vi "Default Instrument Setup.vi"(8 "error in (no error)":errorcluster, 11 "VISA resource name":refnum<visa-resource-name>) -> (0 "error out":errorcluster, 3 "VISA resource name out":refnum<visa-resource-name>)   [LabVIEW 2016, in "Andeen-Hagerling 2700.lvlib"]
doc: "This Utility VI sends a default command string to the instrument whenever a new VISA session is opened, or the instrument is reset. Use this VI as a subVI for the Initialize and Reset VIs. Altering this VI could cause these two VIs to operate incorrectly.\n\nThis VI configures the bridge for performing programmatic control. This includes turning off serial echo, labels, and setting error messages to numeric code, and turning on the Sample Swtich field."
uses:
  Andeen-Hagerling 2700.lvlib
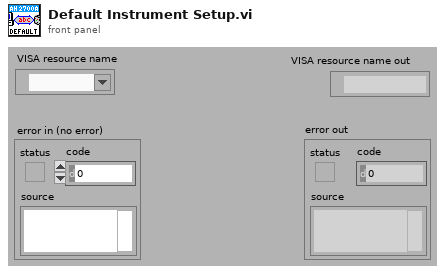
[diagram p1: front panel]
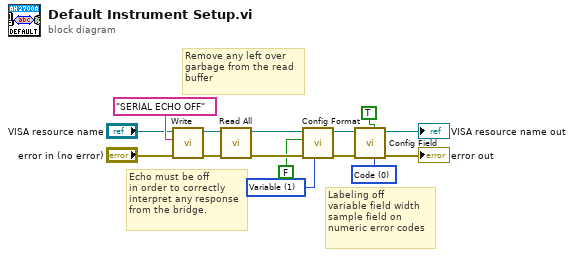
[diagram p0: block diagram]
diagram:
  w1 = 0 items=["Code", "Message"] ("Error Messages (Message)")
  w7 = u16 1 items=["Fixed", "Variable"] ("Field Width (fixed)")
  # "Labeling off\nvariable field width\nsample field on\nnumeric error codes"
  # "Echo must be off\nin order to correctly\ninterpret any response\nfrom the bridge."
  # "Remove any left over\ngarbage from the read\nbuffer"
  n1 = call "Write.vi"("error in"="error in (no error)", "command"="SERIAL ECHO OFF", "VISA resource name"="VISA resource name") -> ("error out"=w11:errorcluster, "VISA resource name out"=w12:refnum<visa-resource-name>)  [unwired: 7 in]
  n2 = call "Read All.vi"("error in"=w11, "VISA resource name"=w12) -> ("error out"=w9:errorcluster, "VISA resource name out"=w10:refnum<visa-resource-name>)  [unwired: 6 in, 2 out]
  n3 = call "Config Format.vi"("Field Width (fixed)"=w7, "error in"=w9, "Labelling (on)"=FALSE, "VISA resource name"=w10) -> ("error out"=w5:errorcluster, "VISA resource name out"=w6:refnum<visa-resource-name>)  [unwired: 6 in]
  n4 = call "Config Field.vi"("Error Messages (Message)"=w1, "Sample (off)"=TRUE, "error in"=w5, "VISA resource name"=w6) -> ("error out"=→"error out":errorcluster, "VISA resource name out"=→"VISA resource name out":refnum<visa-resource-name>)  [unwired: 6 in]
